vi "Default Instrument Setup.vi"(8 "error in (no error)":errorcluster, 10 "Set Defaults? (F)":bool, 11 "VISA resource name":refnum<visa-resource-name>) -> (0 "error out":errorcluster, 3 "VISA resource name out":refnum<visa-resource-name>)   [LabVIEW 2011, in "MGC647C.lvlib"]
doc: "This Utility VI sends a default command string to the instrument whenever a new VISA session is opened, or the instrument is reset. Use this VI as a subVI for the Initialize and Reset VIs. Altering this VI could cause these two VIs to operate incorrectly."
uses:
  <instrlib>/MGC647C/MGC647C.lvlib
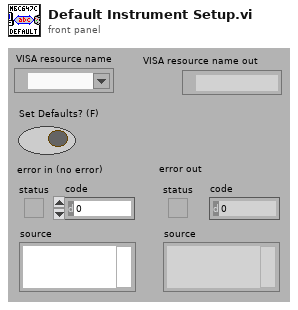
[diagram p1: front panel]
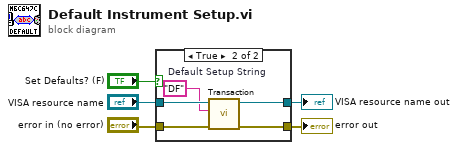
[diagram p0: block diagram]
diagram:
  n1 = case shown="True" "Set Defaults? (F)" {
    tunnel: "VISA resource name" -> [w7 w12]
    tunnel: "error in (no error)" -> [w6 w11]
    tunnel: [w6 w10] -> w3
    tunnel: [w7 w9] -> w2
    frame False {
    }
    frame True {
      w8 = "DF"  # Default Setup String
      n2 = call <instrlib>:"Transaction.vi"("Error In"=w11, "Command"=w8, "VISA resource name"=w12) -> ("Error Out"=w10:errorcluster, "dup VISA resource name"=w9:refnum<visa-resource-name>)  [unwired: 6 in, 1 out]
    }
  }
  "error out" <- w3
  "VISA resource name out" <- w2
